vi "sendEvent.vi"(8 "error in (no error)":errorcluster, 9 "evt_details":cluster{"state":i32}, 10 "evtName":string="event3", 11 "TcpServer in":refnum<class "TcpServer.lvclass">) -> (0 "error out":errorcluster, 3 "TcpServer out":refnum<class "TcpServer.lvclass">)   [LabVIEW 2018, in "TcpServer.lvclass"]
doc: "Send an Event to the Tcp Client."
uses:
  TcpServer.lvclass
  eventTypeDef.ctl
  TcpServer.lvclass/TcpServer.ctl
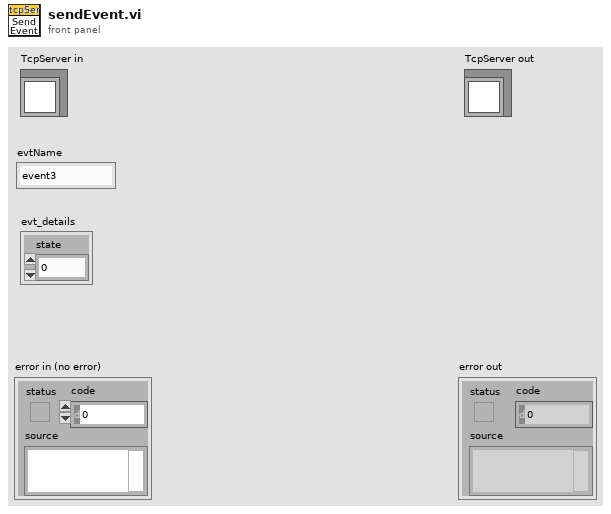
[diagram p1: front panel]
types:
  T1 = typedef "TcpServer.lvclass/eventTypeDef.ctl" = cluster{"evtName":string, "evt_details":cluster{"state":i32}}
  T2 = typedef "TcpServer.lvclass/userEventsTypeDef.ctl" = cluster{"TcpServer":refnum<user-event>, "Command":refnum<user-event>, "Ack":refnum<user-event>, "Event":refnum<user-event>, "Telemetry":refnum<user-event>}
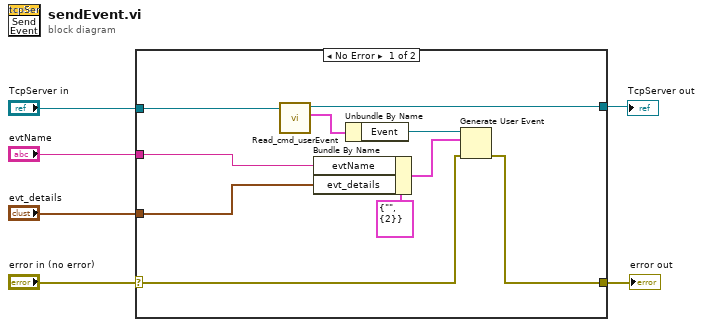
[diagram p0: block diagram]
diagram:
  n1 = case shown="No Error" "error in (no error)" {
    selector: "error in (no error)" -> [w7 w18]
    tunnel: [w8 w18] -> w5
    tunnel: "TcpServer in" -> [w13 w17]
    tunnel: "evtName" -> [w11 _]
    tunnel: "evt_details" -> [w10 _]
    tunnel: [w9 w17] -> w1
    frame No Error {
      n2 = call "Read_cmd_userEvent.vi"("tcpServer in"=w13) -> ("UserEvents"=w12:T2, "tcpServer out"=w9:refnum<class "TcpServer.lvclass">)  [unwired: 8 in, 1 out]
      n3 = Bundle By Name(cluster=T1 {"evtName"="", "evt_details"={"state"=2}}, "evtName"=w11, "evt_details"=w10) -> (w14:T1)
      n4 = Unbundle By Name(w12) -> ("Event"=w16:refnum<user-event>)
      n5 = Generate User Event(user event=w16, event data cluster=w14, error in=w7) -> (error out=w8:errorcluster)  [unwired: 1 in, 1 out]
    }
    frame Error {
    }
  }
  "error out" <- w5
  "TcpServer out" <- w1
